vi "niUSRP Rx Continuous Lab copy.vi"() -> ()   [LabVIEW 2014]
uses:
  <instrlib>/niUSRP/niUSRP Fetch Rx Data (CDB).vi
panel:
  out "Waveform Graph":dbl[](graph)
  out "IQ Plot":dbl[](graph)
  in  "Stop Button":bool
  in  "device name":refnum<k15>="192.168.10.2"
  in  "Active Antenna":string(combo)="RX1"
  in  "samples / frame":i64=1000
  out "Error Out":errorcluster
  out "Gain [dB] (actual)":dbl format="%#.6p"
  out "Carrier Frequency \n[Hz] (actual)":dbl=2450000000.0 format="%#.6p"
  out "IQ Sampling\nRate [s/sec] (actual)":dbl=10000000.0 format="%#.6p"
  in  "Gain [dB]":dbl format="%#.6p"
  in  "Carrier\nFrequency [Hz]":dbl=915000000.0 format="%#.6p"
  in  "IQ Sampling\nRate [s/sec]":dbl=10000000.0 format="%#.6p"
  # "IQ Receiver"
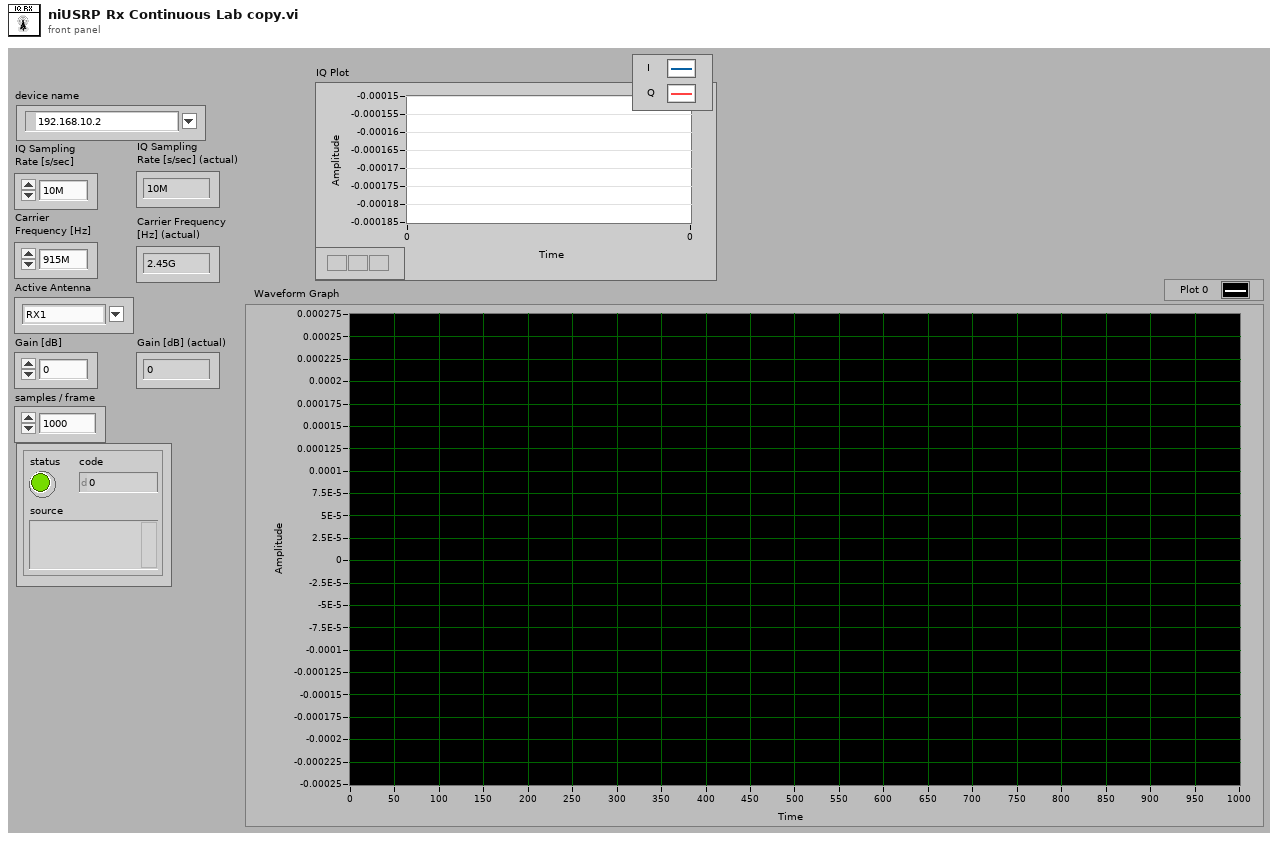
[diagram p1: front panel]
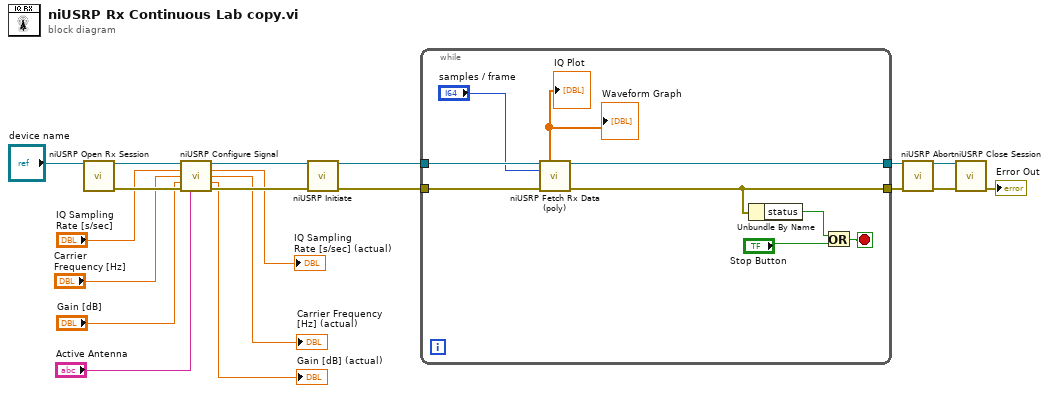
[diagram p0: block diagram]
diagram:
  n1 = call <instrlib>:"niUSRP Open Rx Session.vi"("device names"="device name") -> ("session handle out"=w18:refnum<k15>, "error out"=w17:errorcluster)  [unwired: 13 in]
  n2 = call <instrlib>:"niUSRP Configure Signal.vi"("session handle"=w18, "IQ rate"="IQ Sampling\nRate [s/sec]", "carrier frequency"="Carrier\nFrequency [Hz]", "gain"="Gain [dB]", "error in (no error)"=w17, "active antenna"="Active Antenna") -> ("session handle out"=w7:refnum<k15>, "coerced IQ rate"=→"IQ Sampling\nRate [s/sec] (actual)":dbl, "coerced carrier frequency"=→"Carrier Frequency \n[Hz] (actual)":dbl, "coerced gain"=→"Gain [dB] (actual)":dbl, "error out"=w9:errorcluster)  [unwired: 5 in]
  n3 = call <instrlib>:"niUSRP Initiate.vi"("session handle"=w7, "error in (no error)"=w9) -> ("session handle out"=w13:refnum<k15>, "error out"=w12:errorcluster)  [unwired: 12 in]
  n4 = while {
    tunnel: w13 -> [w28]
    tunnel: w12 -> [w27]
    tunnel: [w24] -> w2
    tunnel: [w23] -> w1
    stop <- w22 stop-if-true
    n5 = call-poly <instrlib>:"niUSRP Fetch Rx Data (poly).vi"("session handle"=w28, "number of samples"="samples / frame", "error in (no error)"=w27) -> ("session handle out"=w24:refnum<k15>, "data"=→"IQ Plot" →"Waveform Graph":cdb[], "error out"=w23:errorcluster)  [unwired: 9 in, 1 out]
    n6 = Unbundle By Name(w23) -> ("status"=w26:bool)
    n7 = Or(x=w26, y="Stop Button") -> (x .or. y?=w22:bool)
  }
  n8 = call <instrlib>:"niUSRP Abort.vi"("session handle"=w2, "error in (no error)"=w1) -> ("session handle out"=w15:refnum<k15>, "error out"=w14:errorcluster)  [unwired: 12 in]
  n9 = call <instrlib>:"niUSRP Close Session.vi"("session handle"=w15, "error in (no error)"=w14) -> ("error out"=→"Error Out":errorcluster)  [unwired: 13 in]
